vi "Configure Standard Waveform.vi"(0 "VISA resource name":refnum<visa-resource-name>, 1 "Frequency (1000 Hz)":dbl[unit]=1000.0, 5 "Channel (0: Channel 1)":T1 items=["Channel 1", "Channel 2"], 7 "Waveform Function (0: Sine)":u16(ring) items=["Sine", "Square", "Pulse", "Ramp", "Noise", "DC", "Sin(x)/x", "Gaussian", "Lorentz", "Exponential Rise", "Exponential Decay", "Haversine"], 9 "Amplitude (1 Vpp)":dbl[unit]=1.0, 11 "error in (no error)":errorcluster, 12 "DC Offset (0.00 V)":dbl[unit]) -> (4 "VISA resource name out":refnum<visa-resource-name>, 15 "error out":errorcluster)   [LabVIEW 2009, in "Tektronix AFG 3000 Series.lvlib"]
doc: "Selects the waveform shape, frequency, amplitude, offset, and phase \nfor a standard waveform."
uses:
  Tektronix AFG 3000 Series.lvlib
  controls.llb/Channel.ctl
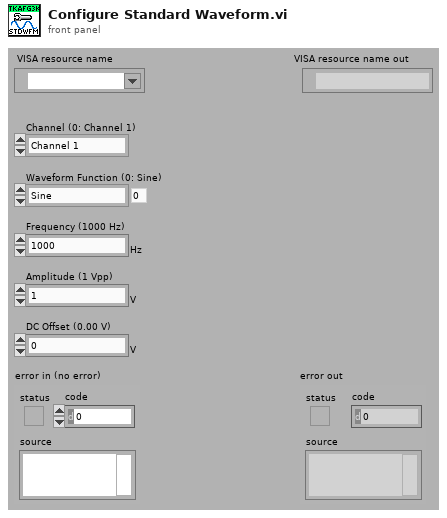
[diagram p1: front panel]
types:
  T1 = typedef "Channel.ctl" = u16
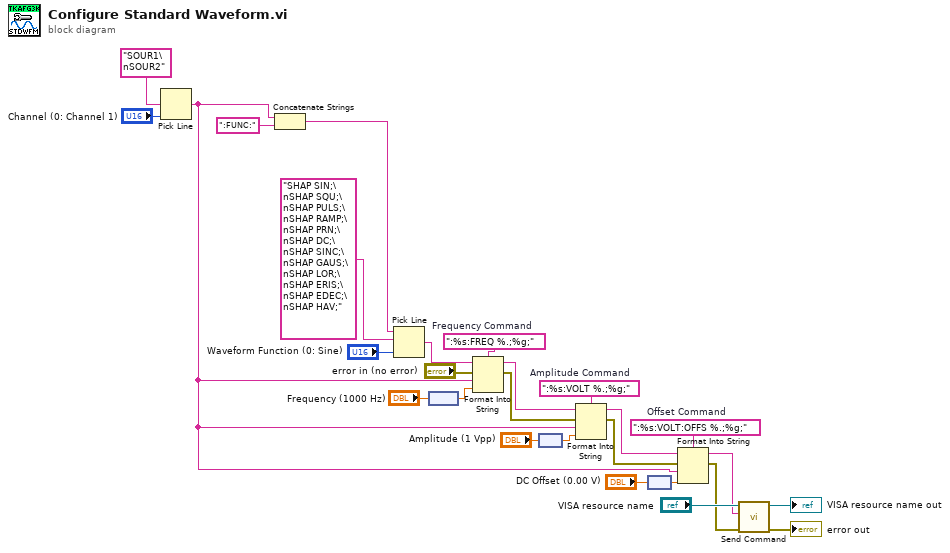
[diagram p0: block diagram]
diagram:
  w22 = ":%s:VOLT:OFFS %.;%g;"  # Offset Command
  w23 = ":%s:VOLT %.;%g;"  # Amplitude Command
  w25 = ":%s:FREQ %.;%g;"  # Frequency Command
  n1 = Pick Line(multi-line string="SOUR1\nSOUR2" ("string (\"\")"), line index="Channel (0: Channel 1)") -> (output string=w15:string)  [unwired: 1 out]
  n2 = Concatenate Strings(w15, ":FUNC:" ("string")) -> (w16:string)
  n3 = Pick Line(string ("")=w16, multi-line string="SHAP SIN;\nSHAP SQU;\nSHAP PULS;\nSHAP RAMP;\nSHAP PRN;\nSHAP DC;\nSHAP SINC;\nSHAP GAUS;\nSHAP LOR;\nSHAP ERIS;\nSHAP EDEC;\nSHAP HAV;" ("Function Command"), line index="Waveform Function (0: Sine)") -> (output string=w24:string)
  n4 = node("Frequency (1000 Hz)") -> (w6:dbl)
  n5 = Format Into String(format string=w25, initial string=w24, error in="error in (no error)", w15, w6) -> (resulting string=w20:string, error out=w13:errorcluster)
  n6 = node("Amplitude (1 Vpp)") -> (w8:dbl)
  n7 = Format Into String(format string=w23, initial string=w20, error in=w13, w15, w8) -> (resulting string=w21:string, error out=w12:errorcluster)
  n8 = node("DC Offset (0.00 V)") -> (w10:dbl)
  n9 = Format Into String(format string=w22, initial string=w21, error in=w12, w15, w10) -> (resulting string=w1:string, error out=w2:errorcluster)
  n10 = call "Send Command.vi"("error in (no error)"=w2, "write buffer"=w1, "VISA resource name"="VISA resource name") -> ("error out"=→"error out":errorcluster, "VISA resource name out"=→"VISA resource name out":refnum<visa-resource-name>)  [unwired: 7 out]
